vi "Write.vi"() -> ()   [LabVIEW 2020]
panel:
  in  "stop":bool
  out "Alarma":bool
  in  "Lim":dbl
  in  "Temp":dbl(slide) scale=0.0..30.0
  out "Gráfica de la señal":dynamicdata(graph)
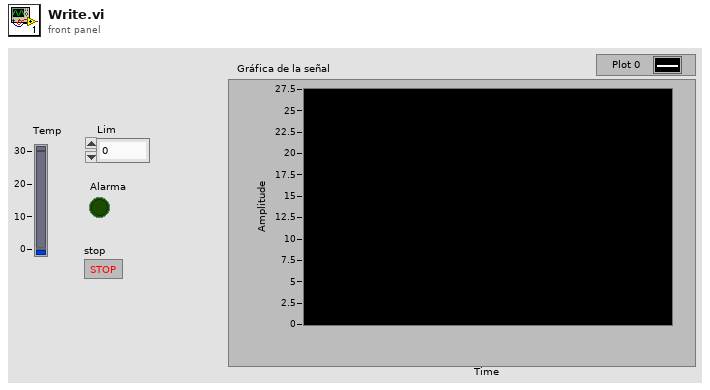
[diagram p1: front panel]
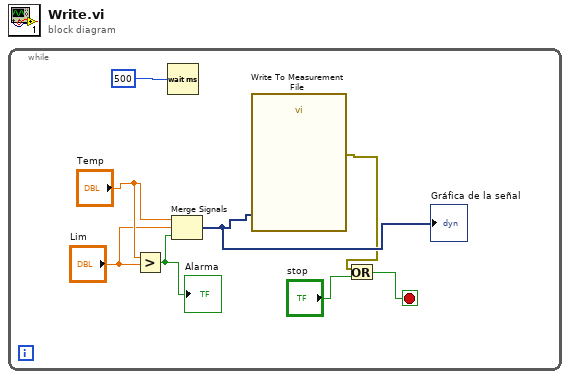
[diagram p0: block diagram]
diagram:
  n1 = while {
    stop <- w2 stop-if-true
    n2 = Greater?(x="Temp", y="Lim") -> (0:w6:bool)
    "Alarma" <- w6
    n3 = Wait (ms)(milliseconds to wait=u32 500) -> ()  [unwired: 1 out]
    n4 = Merge Signals("Temp", "Lim", w6) -> (w4:dynamicdata)
    "Gráfica de la señal" <- w4
    n5 = call "Write To Measurement File"("Signals"=w4) -> ("error out"=w1:errorcluster)  [unwired: 16 in, 2 out]
    n6 = Or(x=w1, y="stop") -> (x .or. y?=w2:bool)
  }
